vi "TagCreatePixelArray.vi"(5 "Layout":string, 7 "Codes":i64[](array[numeric]), 8 "error in (no error)":errorcluster, 11 "ID":i32) -> (0 "error out":errorcluster, 1 "Alpha":u8[][](array[numeric]), 3 "Pixels":u8[][](array[numeric]))   [LabVIEW 2020, in "g_ar_toolkit.feature_detection.lvlib"]
uses:
  g_ar_toolkit.feature_detection.lvlib
  TagPixelType.ctl
  <vilib>/Utility/error.llb/Error Cluster From Error Code.vi
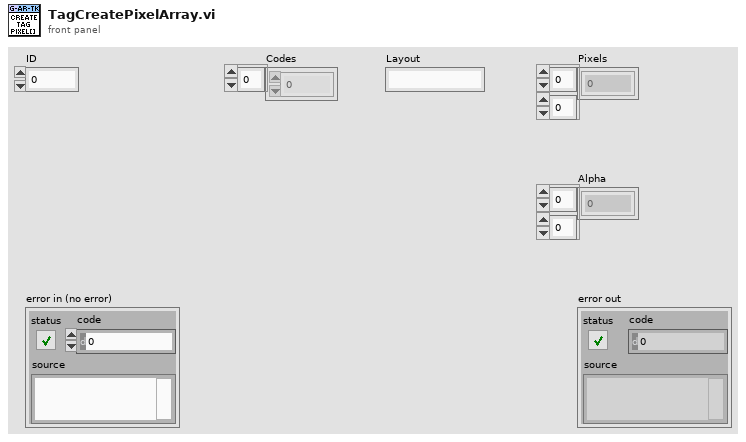
[diagram p1: front panel]
types:
  T1 = typedef "g_ar_toolkit.feature_detection.lvlib/TagPixelType.ctl" = enum8{"Black", "White", "Transparent"}
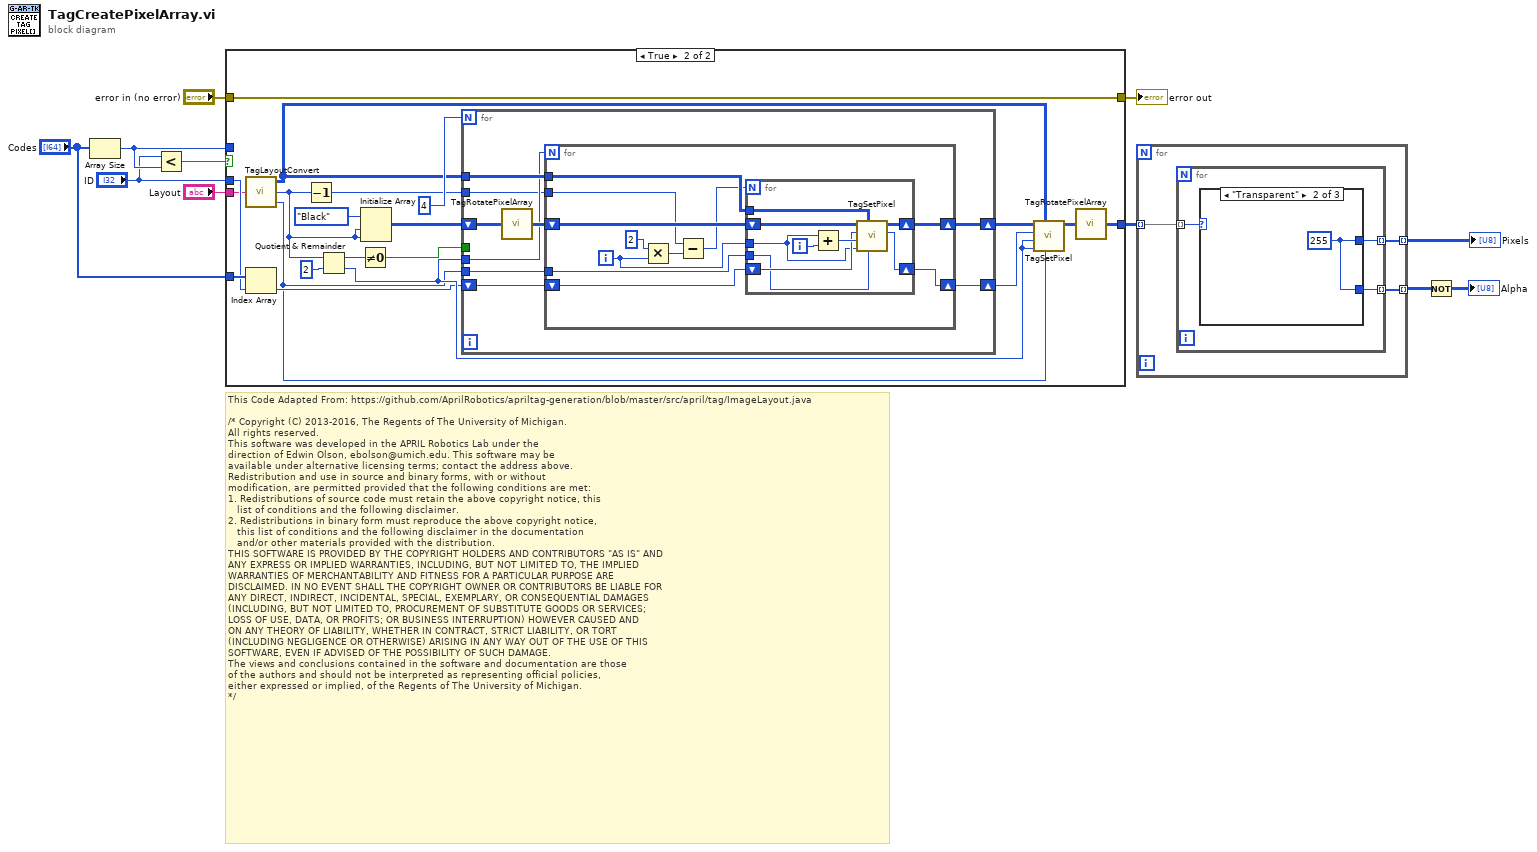
[diagram p0: block diagram]
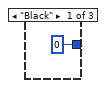
[diagram p2: hidden frame]
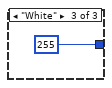
[diagram p3: hidden frame]
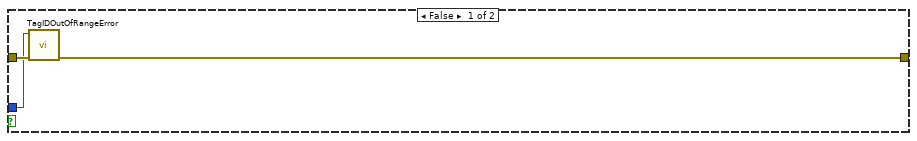
[diagram p4: hidden frame]
diagram:
  # "This Code Adapted From: https://github.com/AprilRobotics/apriltag-generation/blob/master/src/april/tag/ImageLayout.java\n\n/* Copyright (C) 2013-2016, The Regents of The University of Michigan.\nAll rights reserved.\nThis software was developed in the APRIL Robotics Lab under the\ndirection of Edwin Olson, ebolson@umich.edu. This software may be\navailable under alternative licensing terms; contact the address above.\nRedistribution and use in source and binary forms, with or without\nmodification, are permitted provided that the following conditions are met:\n1. Redistributions of source code must retain the above copyright notice, this\n   list of conditions and the following disclaimer.\n2. Redistributions in binary form must reproduce the above copyright notice,\n   this list of conditions and the following disclaimer in the documentation\n   and/or other materials provided with the distribution.\nTHIS SOFTWARE IS PROVIDED BY THE COPYRIGHT HOLDERS AND CONTRIBUTORS \"AS IS\" AND\nANY EXPRESS OR IMPLIED WARRANTIES, INCLUDING, BUT NOT LIMITED TO, THE IMPLIED\nWARRANTIES OF MERCHANTABILITY AND FITNESS FOR A PARTICULAR PURPOSE ARE\nDISCLAIMED. IN NO EVENT SHALL THE COPYRIGHT OWNER OR CONTRIBUTORS BE LIABLE FOR\nANY DIRECT, INDIRECT, INCIDENTAL, SPECIAL, EXEMPLARY, OR CONSEQUENTIAL DAMAGES\n(INCLUDING, BUT NOT LIMITED TO, PROCUREMENT OF SUBSTITUTE GOODS OR SERVICES;\nLOSS OF USE, DATA, OR PROFITS; OR BUSINESS INTERRUPTION) HOWEVER CAUSED AND\nON ANY THEORY OF LIABILITY, WHETHER IN CONTRACT, STRICT LIABILITY, OR TORT\n(INCLUDING NEGLIGENCE OR OTHERWISE) ARISING IN ANY WAY OUT OF THE USE OF THIS\nSOFTWARE, EVEN IF ADVISED OF THE POSSIBILITY OF SUCH DAMAGE.\nThe views and conclusions contained in the software and documentation are those\nof the authors and should not be interpreted as representing official policies,\neither expressed or implied, of the Regents of The University of Michigan.\n*/"
  n1 = Array Size(array="Codes") -> (size(s)=w10:i32)
  n2 = Less?(x="ID", y=w10) -> (x < y?=w7:bool)
  n3 = case shown="True" w7 {
    tunnel: "Codes" -> [_ w34]
    tunnel: "ID" -> [_ w33]
    tunnel: "error in (no error)" -> [w14 w16]
    tunnel: [w13 w16] -> w9
    tunnel: w10 -> [w12 _]
    tunnel: "Layout" -> [_ w20]
    tunnel: [_ w21] -> w4
    frame False {
      n4 = call "TagIDOutOfRangeError.vi"("error in (no error)"=w14, "Tag Family Size"=w12) -> ("error out"=w13:errorcluster)  [unwired: 9 in]
    }
    frame True {
      n5 = call "TagLayoutConvert.vi"("Layout"=w20) -> ("Pixel Map"=w19:u8[][], "Size"=w17:i32, "Number Of Bits"=w18:i32)
      n6 = Index Array(array=w34, index=w33) -> (element=w22:i64)
      n7 = Decrement(x=w17) -> (x-1=w25:i32)
      n8 = Quotient & Remainder(x=w17, y=2) -> (x-y*floor(x/y)=w24:i32, floor(x/y)=w26:i32)
      n9 = Not Equal To 0?(x=w24) -> (x != 0?=w29:bool)
      n10 = Initialize Array(TagPixelType."Black", w17, w17) -> (w15:T1[][])
      n11 = for {
        N: 4 -> [_]
        shift-right: [w39] -> w30
        shift-left: w15 -> [w41]
        tunnel: w26 -> [w36]
        tunnel: w25 -> [w35]
        tunnel: w19 -> [w43]
        tunnel: w18 -> [w42]
        tunnel: w29 -> [_]
        shift-right: [w37] -> w32
        shift-left: w22 -> [w38]
        n12 = call "TagRotatePixelArray.vi"("Pixel Array In"=w41) -> ("Rotated Pixel Array"=w40:T1[][])
        n13 = for {
          N: w36 -> [_]
          tunnel: w43 -> [w54]
          shift-right: [w52] -> w39
          shift-left: w40 -> [w53]
          tunnel: w42 -> [w51]
          shift-right: [w49] -> w37
          shift-left: w38 -> [w50]
          tunnel: w35 -> [w47]
          i -> [w48]
          n14 = Multiply(x=2, y=w48) -> (x*y=w46:i32)
          n15 = Subtract(x=w47, y=w46) -> (x-y=w44:i32)
          n16 = for {
            N: w44 -> [_]
            tunnel: w48 -> [w56]
            tunnel: w54 -> [w58]
            shift-right: [w62] -> w52
            shift-left: w53 -> [w60]
            tunnel: w51 -> [w55]
            shift-right: [w61] -> w49
            shift-left: w50 -> [w57]
            i -> [w63]
            n17 = Add(x=w56, y=w63) -> (x+y=w59:i32)
            n18 = call "TagSetPixel.vi"("Number of Bits"=w55, "Pixel Type Map"=w58, "y"=w56, "x"=w59, "Code in"=w57, "Pixels in"=w60) -> ("Code out"=w61:i64, "Pixels out"=w62:T1[][])  [unwired: 4 in]
          }
        }
      }
      n19 = call "TagSetPixel.vi"("Number of Bits"=w18, "Pixel Type Map"=w19, "y"=w26, "x"=w26, "Code in"=w32, "Pixels in"=w30) -> ("Pixels out"=w31:T1[][])  [unwired: 4 in, 1 out]
      n20 = call "TagRotatePixelArray.vi"("Pixel Array In"=w31) -> ("Rotated Pixel Array"=w21:T1[][])
    }
  }
  "error out" <- w9
  n21 = for {
    tunnel: w4 -> [w66] mode=indexing
    tunnel: [w65] -> w1 mode=indexing
    tunnel: [w64] -> w3 mode=indexing
    n22 = for {
      tunnel: w66 -> [w69] mode=indexing
      tunnel: [w68] -> w65 mode=indexing
      tunnel: [w67] -> w64 mode=indexing
      n23 = case shown="\"Transparent\"" w69 {
        tunnel: [u8 0 w71 u8 255] -> w68
        tunnel: [_ w71 _] -> w67
        frame "Black" {
        }
        frame "Transparent" {
          w71 = u8 255
        }
        frame "White" {
        }
      }
    }
  }
  "Pixels" <- w1
  n24 = Not(x=w3) -> (.not. x?=→"Alpha":u8[][])
